vi "Turn Note Event into Boolean.vi"(11 "element":T1) -> (3 "Boolean array":bool[](array[boolean]))   [LabVIEW 2016]
uses:
  Notes.ctl
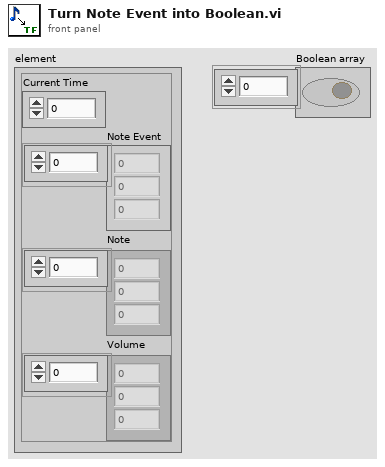
[diagram p1: front panel]
types:
  T1 = typedef "Notes.ctl" = cluster{"Current Time":u32, "Note Event":u32[], "Note":u32[], "Volume":u32[]}
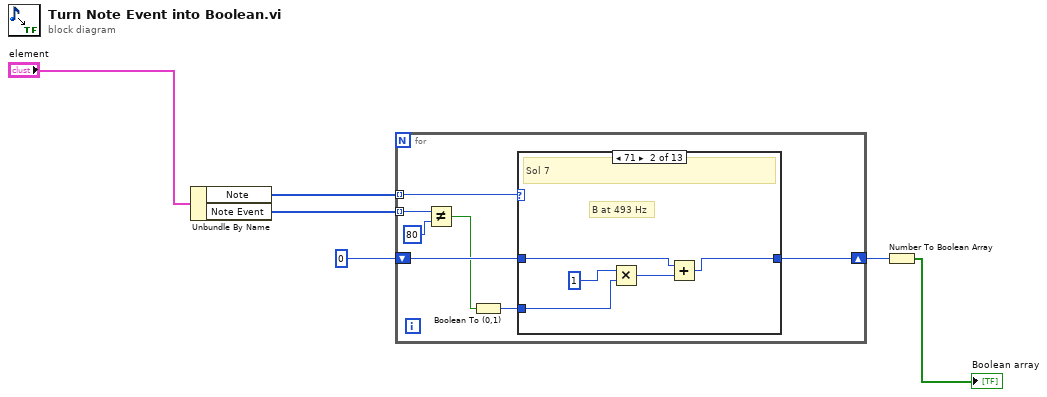
[diagram p0: block diagram]
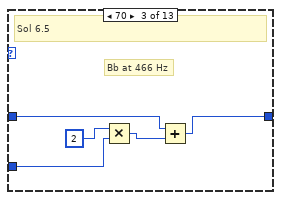
[diagram p3: hidden frame]
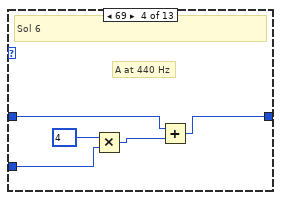
[diagram p4: hidden frame]
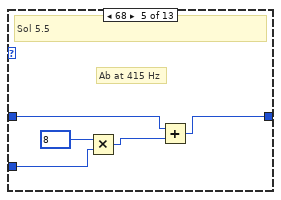
[diagram p5: hidden frame]
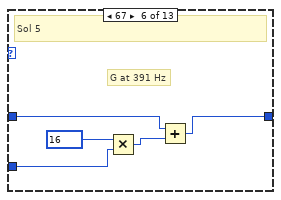
[diagram p6: hidden frame]
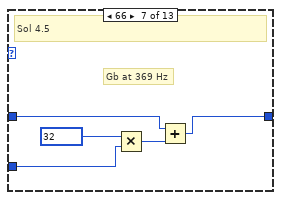
[diagram p7: hidden frame]
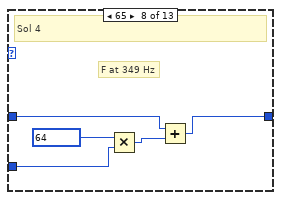
[diagram p8: hidden frame]
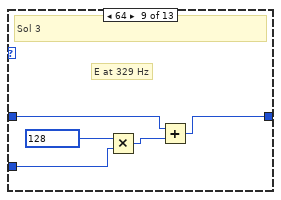
[diagram p9: hidden frame]
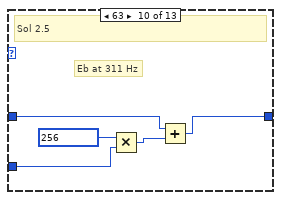
[diagram p10: hidden frame]
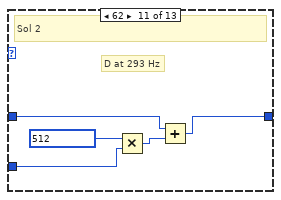
[diagram p11: hidden frame]
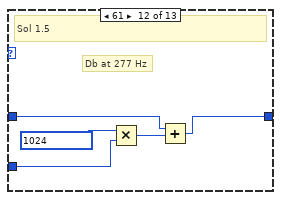
[diagram p12: hidden frame]
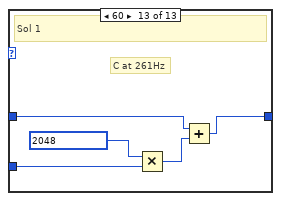
[diagram p13: hidden frame]
diagram:
  n1 = Unbundle By Name("element") -> ("Note"=w4:u32[], "Note Event"=w5:u32[])
  n2 = for {
    shift-right: [w13] -> w2
    shift-left: 0 -> [w12]
    tunnel: w4 -> [w11] mode=indexing
    tunnel: w5 -> [w10] mode=indexing
    n3 = Not Equal?(x=w10, y=u32 80) -> (x != y?=w7:bool)
    n4 = Boolean To (0,1)(Boolean=w7) -> (0, 1=w8:i16)
    n5 = case shown="71" w11 {
      tunnel: [w14 w17 w22 w27 w32 w37 w42 w47 w52 w57 w62 w67 w73] -> w13
      tunnel: w12 -> [w14 w18 w23 w28 w33 w38 w43 w48 w53 w58 w63 w68 w74]
      tunnel: w8 -> [_ w15 w20 w25 w30 w35 w40 w45 w50 w55 w60 w65 w70]
      frame 0, Default {
      }
      frame 71 {
        # "B at 493 Hz"
        # "Sol 7"
        n6 = Multiply(x=1, y=w15) -> (x*y=w16:i32)
        n7 = Add(x=w18, y=w16) -> (x+y=w17:u32)
      }
      frame 70 {
        # "Bb at 466 Hz"
        # "Sol 6.5"
        n8 = Multiply(x=2, y=w20) -> (x*y=w21:i32)
        n9 = Add(x=w23, y=w21) -> (x+y=w22:u32)
      }
      frame 69 {
        # "A at 440 Hz"
        # "Sol 6"
        n10 = Multiply(x=4, y=w25) -> (x*y=w26:i32)
        n11 = Add(x=w28, y=w26) -> (x+y=w27:u32)
      }
      frame 68 {
        # "Ab at 415 Hz"
        # "Sol 5.5"
        n12 = Multiply(x=8, y=w30) -> (x*y=w31:i32)
        n13 = Add(x=w33, y=w31) -> (x+y=w32:u32)
      }
      frame 67 {
        # "G at 391 Hz"
        # "Sol 5"
        n14 = Multiply(x=16, y=w35) -> (x*y=w36:i32)
        n15 = Add(x=w38, y=w36) -> (x+y=w37:u32)
      }
      frame 66 {
        # "Gb at 369 Hz"
        # "Sol 4.5"
        n16 = Multiply(x=32, y=w40) -> (x*y=w41:i32)
        n17 = Add(x=w43, y=w41) -> (x+y=w42:u32)
      }
      frame 65 {
        # "F at 349 Hz"
        # "Sol 4"
        n18 = Multiply(x=64, y=w45) -> (x*y=w46:i32)
        n19 = Add(x=w48, y=w46) -> (x+y=w47:u32)
      }
      frame 64 {
        # "E at 329 Hz"
        # "Sol 3"
        n20 = Multiply(x=128, y=w50) -> (x*y=w51:i32)
        n21 = Add(x=w53, y=w51) -> (x+y=w52:u32)
      }
      frame 63 {
        # "Eb at 311 Hz"
        # "Sol 2.5"
        n22 = Multiply(x=256, y=w55) -> (x*y=w56:i32)
        n23 = Add(x=w58, y=w56) -> (x+y=w57:u32)
      }
      frame 62 {
        # "D at 293 Hz"
        # "Sol 2"
        n24 = Multiply(x=512, y=w60) -> (x*y=w61:i32)
        n25 = Add(x=w63, y=w61) -> (x+y=w62:u32)
      }
      frame 61 {
        # "Db at 277 Hz"
        # "Sol 1.5"
        n26 = Multiply(x=1024, y=w65) -> (x*y=w66:i32)
        n27 = Add(x=w68, y=w66) -> (x+y=w67:u32)
      }
      frame 60 {
        # "C at 261Hz"
        # "Sol 1"
        n28 = Multiply(x=u32 2048, y=w70) -> (x*y=w72:u32)
        n29 = Add(x=w74, y=w72) -> (x+y=w73:u32)
      }
    }
  }
  n30 = Number To Boolean Array(number=w2) -> (Boolean array=→"Boolean array":bool[])
